vi "Destroy Semaphore(8.5).vi"(4 "error in (no error)":errorcluster, 7 "semaphore":T1) -> (0 "error out":errorcluster, 3 "semaphore name":string)   [LabVIEW 2014]
doc: "LabVIEW no longer supports this VI. Use the Release Semaphore Reference VI instead. However, the Embedded Module for ARM Microcontrollers, Embedded Module for Blackfin Processors, Microprocessor SDK, Touch Panel Module, and Windows Mobile Module still support this VI.\n\nDestroys the specified semaphore. All Acquire Semaphore VIs that are currently waiting on this semaphore time out immediately and return an error."
uses:
  <vilib>/Utility/semaphor.llb/Semaphore Name & Ref DB Action.ctl
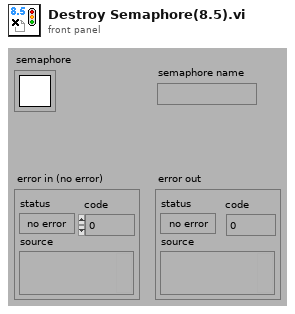
[diagram p1: front panel]
types:
  T1 = typedef "Semaphore RefNum" = refnum<k1>
  T2 = typedef "Semaphore Name & Ref DB Action.ctl" = enum16{"Lookup", "Insert", "Remove"}
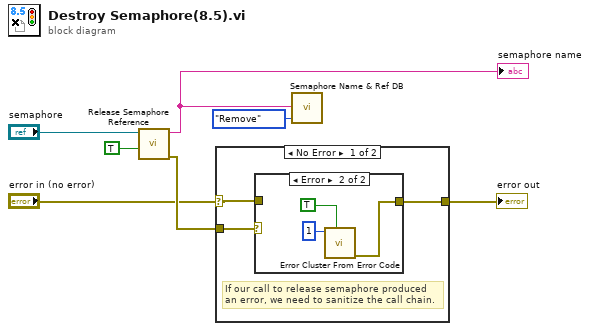
[diagram p0: block diagram]
diagram:
  n1 = call <vilib>:"Release Semaphore Reference.vi"("force destroy? (F)"=TRUE, "semaphore"="semaphore") -> ("error out"=w2:errorcluster, "semaphore name"=w4:string)  [unwired: 1 in, 7 out]
  "semaphore name" <- w4
  n2 = case shown="No Error" "error in (no error)" {
    selector: "error in (no error)" -> [w8 w15]
    tunnel: [w10 w15] -> w3
    tunnel: w2 -> [w9 _]
    frame No Error {
      # "If our call to release semaphore produced an error, we need to sanitize the call chain."
      n3 = case shown="Error" w9 {
        tunnel: [w11 w12] -> w10
        tunnel: w8 -> [w11 _]
        frame No Error {
        }
        frame Error {
          n4 = call <vilib>:"Error Cluster From Error Code.vi"("show call chain? (False)"=TRUE, "error code (0)"=1) -> ("error out"=w12:errorcluster)  [unwired: 1 in, 6 out]
        }
      }
    }
    frame Error {
    }
  }
  "error out" <- w3
  n5 = call <vilib>:"Semaphore Name & Ref DB.vi"("Semaphore Action"=Semaphore_Name_&_Ref_DB_Action."Remove", "Semaphore Name"=w4) -> ()  [unwired: 1 in, 1 out]
